vi "Write Menu selections.vi"(8 "error in (no error)":errorcluster, 10 "Menu selections":string[](array[string]), 11 "Menu object parameters in":refnum<class "Menu object parameters.lvclass">) -> (0 "error out":errorcluster, 3 "Menu object parameters out":refnum<class "Menu object parameters.lvclass">)   [LabVIEW 2015, in "Menu object parameters.lvclass"]
uses:
  Menu object parameters.lvclass
  Menu object parameters.lvclass/Menu object parameters.ctl
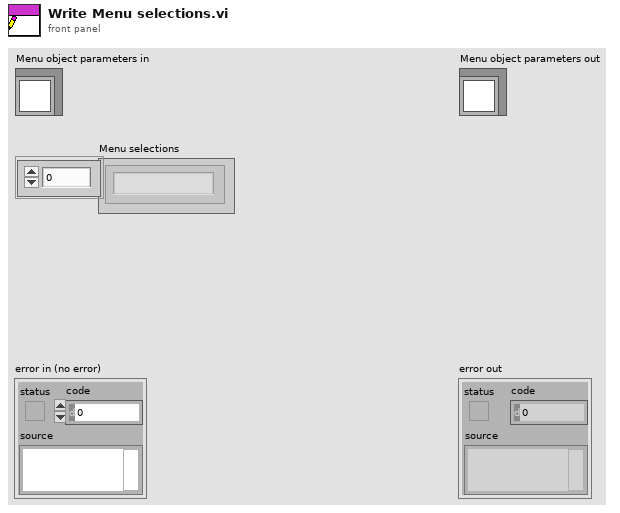
[diagram p1: front panel]
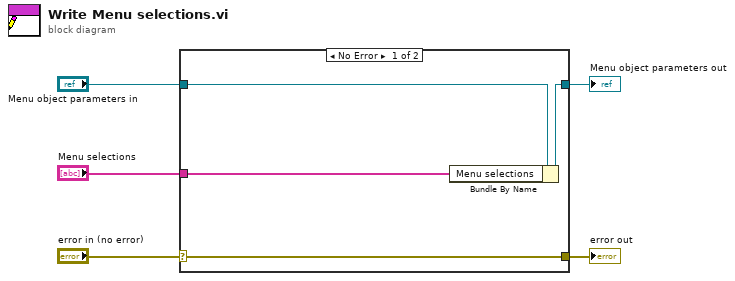
[diagram p0: block diagram]
diagram:
  n1 = case shown="No Error" "error in (no error)" {
    selector: "error in (no error)" -> [w9 w10]
    tunnel: [w9 w10] -> w4
    tunnel: [w7 w11] -> w2
    tunnel: "Menu object parameters in" -> [w8 w11]
    tunnel: "Menu selections" -> [w6 _]
    frame No Error {
      n2 = Bundle By Name(cluster=w8, "Menu selections"=w6) -> (w7:refnum<class "Menu object parameters.lvclass">)
    }
    frame Error {
    }
  }
  "error out" <- w4
  "Menu object parameters out" <- w2
